vi "test usage.vi"() -> ()   [LabVIEW 2009]
panel:
  out "Decoded Data":dbl[](array[numeric]) format="%.2f"
  out "new picture":picture
  in  "address":string="192.168.1.7"
  in  "stop":bool
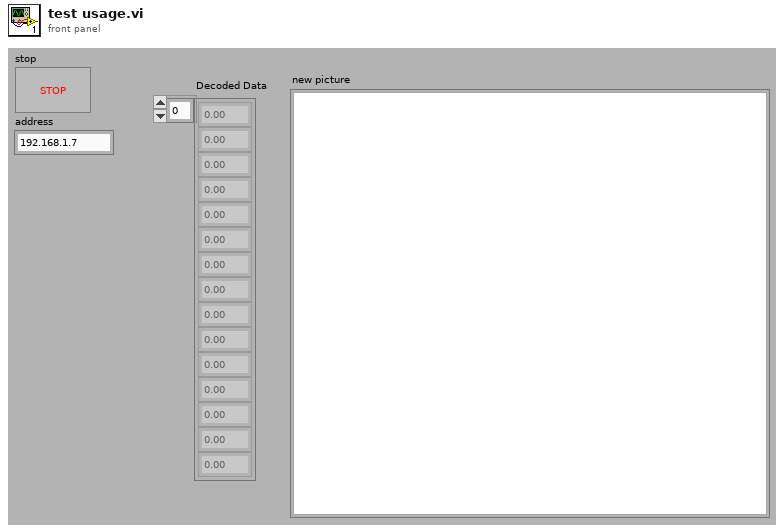
[diagram p1: front panel]
types:
  T1 = typedef "LVBoundsTypeDef.ctl" = cluster{"Width":u32, "Height":u32}
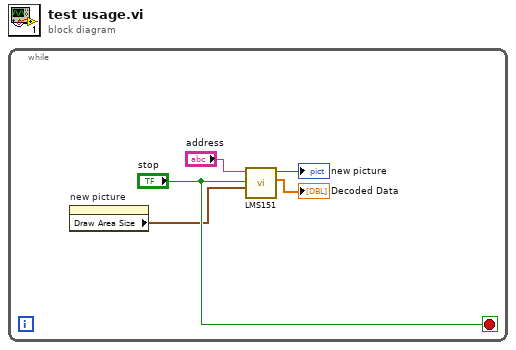
[diagram p0: block diagram]
diagram:
  n1 = while {
    stop <- "stop" stop-if-true
    n2 = property on="new picture" class="Pict"() -> ("Draw Area Size"=w1:T1)  [unwired: 2 in, 2 out]
    n3 = call "LMS151.vi"("Draw Area Size"=w1, "stop"="stop", "address"="address") -> ("Decoded Data"=→"Decoded Data":dbl[], "new picture"=→"new picture":picture)  [unwired: 7 in]
  }
